vi "Create name of exp.vi"(8 "error in (no error)":errorcluster, 10 "Exp name":string, 11 "Control-Client in":refnum<class "Control-Client.lvclass">) -> (0 "error out":errorcluster, 1 "name out":string, 2 "Numeric":i32, 3 "Control-Client out":refnum<class "Control-Client.lvclass">, 4 "Experiments_group out":refnum<class "Experiments_group.lvclass">)   [LabVIEW 2020, in "Control-Client.lvclass"]
uses:
  Control-Client.lvclass
  Experiments/Experiments_group.lvclass
  Control-Client.lvclass/Control-Client.ctl
  Experiments/Experiments_group.lvclass/Experiments_group.ctl
  methods/Read Group #.vi
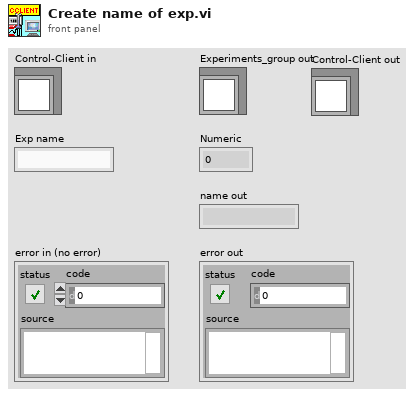
[diagram p1: front panel]
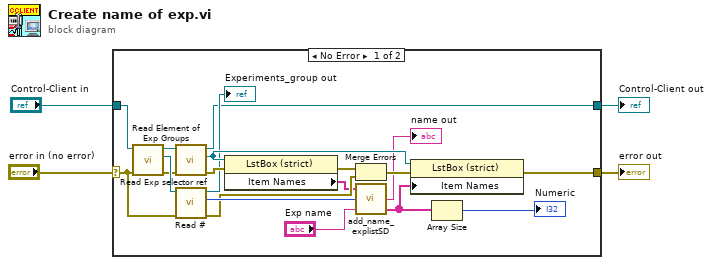
[diagram p0: block diagram]
diagram:
  n1 = case shown="No Error" "error in (no error)" {
    selector: "error in (no error)" -> [w8 w25]
    tunnel: [w23 w25] -> w4
    tunnel: "Control-Client in" -> [w16 w24]
    tunnel: [w6 w24] -> w1
    frame No Error {
      n2 = call "Read Element of Exp Groups.vi"("error in (no error)"=w8, "Control-Client in"=w16) -> ("error out"=w10:errorcluster, "Experiments_group.lvclass"=w20:refnum<class "Experiments_group.lvclass">, "Control-Client out"=w11:refnum<class "Control-Client.lvclass">)  [unwired: 7 in]
      n3 = call "Read Exp selector ref.vi"("error in (no error)"=w10, "Control-Client in"=w11) -> ("error out"=w9:errorcluster, "Exp selector ref"=w14:refnum<vi>, "Control-Client out"=w6:refnum<class "Control-Client.lvclass">)  [unwired: 7 in]
      n4 = call "Read # .vi"("error in (no error)"=w8, "Experiments_group in"=w20) -> ("error out"=w21:errorcluster, "#"=w22:i32, "Experiments_group out"=→"Experiments_group out":refnum<class "Experiments_group.lvclass">)  [unwired: 7 in]
      n5 = property on="Property Node" class="LstBox (strict)"(reference=w14, error in=w9) -> (error out=w5:errorcluster, "Item Names"=w15:string[])  [unwired: 1 out]
      n6 = Merge Errors(w5, w21) -> (w17:errorcluster)
      n7 = call "add_name_explistSD.vi"("Exp name"="Exp name", "#"=w22, "Item Names in"=w15) -> ("Item Names out"=w18:string[], "name out"=→"name out":string)  [unwired: 1 in]
      n8 = property on="Property Node" class="LstBox (strict)"(reference=w14, error in=w17, "Item Names"=w18) -> (error out=w23:errorcluster)  [unwired: 1 out]
      n9 = Array Size(array=w18) -> (size(s)=→"Numeric":i32)
    }
    frame Error {
    }
  }
  "error out" <- w4
  "Control-Client out" <- w1
